vi "refresh enum.vi"(8 "error in (no error)":errorcluster, 11 "LineCCD in":refnum<class "LineCCD.lvclass">) -> (0 "error out":errorcluster, 3 "LineCCD out":refnum<class "LineCCD.lvclass">)   [LabVIEW 2012, in "LineCCD.lvclass"]
uses:
  LineCCD.lvclass
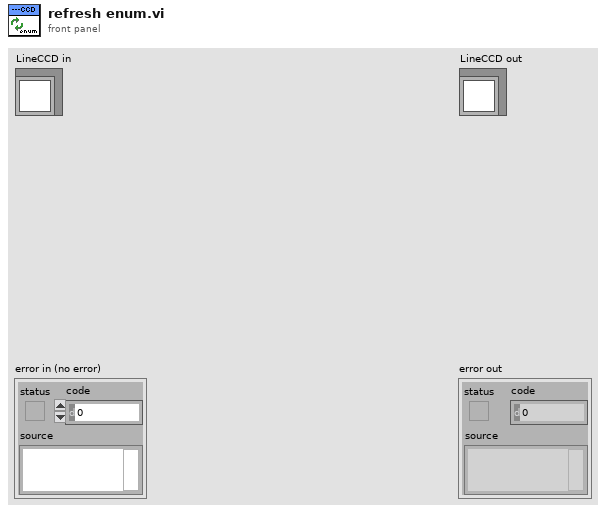
[diagram p1: front panel]
types:
  T1 = typedef "LineCCD.lvclass/Fit ERF.ctl" = enum16{"Default", "derivative 4x", "Fit ERF", "Fit ERF x4"}
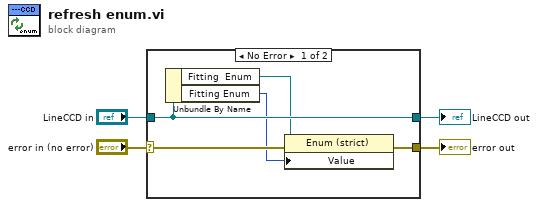
[diagram p0: block diagram]
diagram:
  n1 = case shown="No Error" "error in (no error)" {
    selector: "error in (no error)" -> [w7 w11]
    tunnel: [w6 w11] -> w3
    tunnel: [w9 w10] -> w1
    tunnel: "LineCCD in" -> [w9 w10]
    frame No Error {
      n2 = Unbundle By Name(w9) -> ("Fitting  Enum"=w8:refnum<vi>, "Fitting Enum"=w5:T1)
      n3 = property class="Enum (strict)"(reference=w8, error in=w7, "Value"=w5) -> (error out=w6:errorcluster)  [unwired: 1 out]
    }
    frame Error {
    }
  }
  "error out" <- w3
  "LineCCD out" <- w1
